vi "SV TDMS Read Function Info.vi"(8 "error in (no error)":errorcluster, 9 "channel name":string, 10 "group name":string, 11 "tdms file in":refnum<k34>) -> (0 "error out":errorcluster, 1 "channel name out":string, 2 "group name out":string, 3 "tdms file out":refnum<k34>, 4 "function info":T2 {"function type" items=["Signal"=0, "Speed"=3, "Ratio"=6, "Count"=7, "-"=9, "Level"=10, "-"=19, "Octave Spectrum"=20, "-"=29, "FFT Auto Spectrum"=30, "FFT Cross Spectrum"=40, "Frequency Response"=50, "-"=59, "Event"=90, "None"=98]; "function subtype" items=["Unscaled binary"=0, "Scaled voltage"=1, "Scaled engineering units"=2, "-"=10, "Value"=19, "DC"=11, "AC"=12, "RMS^2"=13, "RMS"=14, "Peak"=15, "Peak to peak"=16, "-"=20, "1/1 octave"=21, "1/3 octave"=22, "1/6 octave"=23, "1/12 octave"=24, "1/24 octave"=25, "-"=30, "Density"=31, "Magnitude"=32, "Phase"=33, "Real"=34, "Imaginary"=35, "Complex"=345, "Coherence"=36, "-"=90, "None"=98, "Unknown"=99]; "X-dimension" items=["Time (s)"=0, "Frequency-CB (Hz)"=1, "Frequency-CPB (Hz)"=1248, "Frequency-Arbitrary (Hz)"=2357, "Quefrency (s)"=2, "Revolutions (rev)"=3, "Order"=4, "Speed (RPM)"=11, "Speed (rad/s)"=21, "Critical Band"=31, "Critical Band Rate (Bark)"=32, "None"=98, "Index"=65535]}, 6 "LabVIEW datatype":T1 items=["String: abc"=7, "Boolean: True or False"=8, "Scalar: y"=0, "Array: Y"=1, "Waveform: t0, dt, Y, variant"=2, "Cluster: x0, dx, Y"=3, "Cluster: X, Y"=4, "Waterfall"=5, "Colormap"=6])   [LabVIEW 2017]
uses:
  <vilib>/addons/_NISVFA/_Shared subVIs/Controls/NI Function Info.ctl
  <vilib>/addons/_NISVFA/_Shared subVIs/Controls/NI Function Type.ctl
  <vilib>/addons/_NISVFA/_Shared subVIs/Controls/NI Function SubType.ctl
  <vilib>/addons/_NISVFA/_Shared subVIs/Controls/svc_X-Axis Units.ctl
  <vilib>/addons/_NISVFA/_Shared subVIs/Controls/LV Datatypes.ctl
  <vilib>/addons/_NISVFA/_Shared subVIs/Controls/NI Channel Properties.ctl
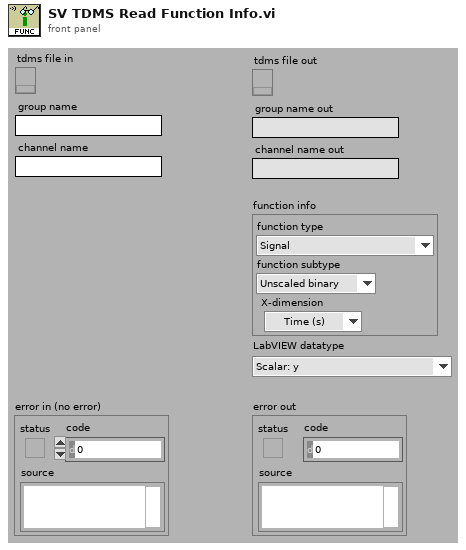
[diagram p1: front panel]
types:
  T1 = typedef "LV Datatypes.ctl" = i32
  T2 = typedef "NI Function Info.ctl" = cluster{"function type":T3, "function subtype":T4, "X-dimension":T5}
  T3 = typedef "NI Function Type.ctl" = u16
  T4 = typedef "NI Function SubType.ctl" = u16
  T5 = typedef "svc_X-Axis Units.ctl" = u16
  T6 = typedef "NI Channel Properties.ctl" = u16
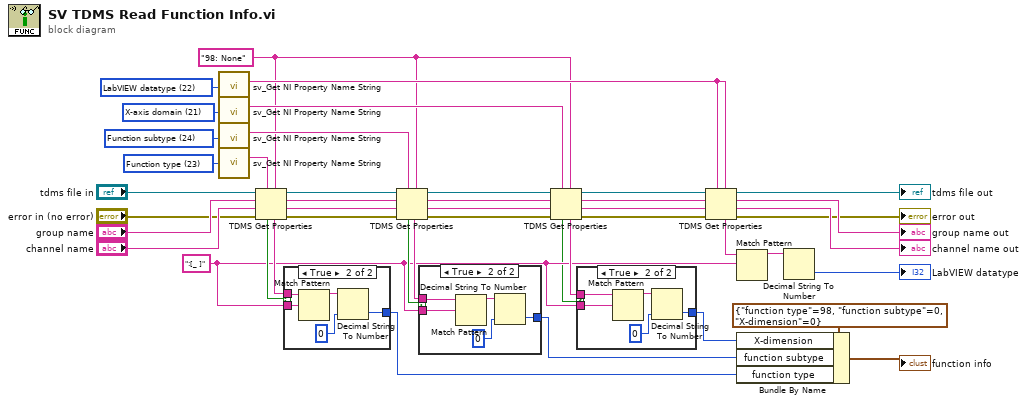
[diagram p0: block diagram]
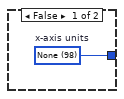
[diagram p2: hidden frame]
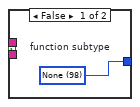
[diagram p3: hidden frame]
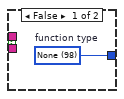
[diagram p4: hidden frame]
diagram:
  w1 = "98: None" ("data type")
  w4 = ":[_ ]" ("regular expression")
  w29 = T6 22 items=["Channel name", "Channel description", "Y-axis label", "Y-axis unit string", "X-axis label", "X-axis unit string", "x0", "dx", "Number of samples", "X channel", "Filter settled", "dB reference", "Window", "Window parameter", "Window size", "FFT size", "Peak units", "Spectrum type", "Magnitude scale", "Spectral density", "Sensor sensitivity (mV/EU)", "X-axis domain", "LabVIEW datatype"] ("property")
  w31 = T6 24 items=["Channel name", "Channel description", "Y-axis label", "Y-axis unit string", "X-axis label", "X-axis unit string", "x0", "dx", "Number of samples", "X channel", "Filter settled", "dB reference", "Window", "Window parameter", "Window size", "FFT size", "Peak units", "Spectrum type", "Magnitude scale", "Spectral density", "Sensor sensitivity (mV/EU)", "X-axis dimension", "LabVIEW datatype", "Function type", "Function subtype"] ("property")
  w32 = T6 21 items=["Channel name", "Channel description", "Y-axis label", "Y-axis unit string", "X-axis label", "X-axis unit string", "x0", "dx", "Number of samples", "X channel", "Filter settled", "dB reference", "Window", "Window parameter", "Window size", "FFT size", "Peak units", "Spectrum type", "Magnitude scale", "Spectral density", "Sensor sensitivity (mV/EU)", "X-axis domain", "LabVIEW datatype", "Function type", "Component", "Level detector"] ("property")
  w30 = T6 23 items=["Channel name", "Channel description", "Y-axis label", "Y-axis unit string", "X-axis label", "X-axis unit string", "x0", "dx", "Number of samples", "X channel", "Filter settled", "dB reference", "Window", "Window parameter", "Window size", "FFT size", "Peak units", "Spectrum type", "Magnitude scale", "Spectral density", "Sensor sensitivity (mV/EU)", "X-axis domain", "LabVIEW datatype", "Function type", "Component", "Level detector"] ("property")
  n1 = call <vilib>:"sv_Get NI Property Name String.vi"("property"=w29) -> ("TDMS property name"=w17:string)  [unwired: 13 in, 1 out]
  n2 = call <vilib>:"sv_Get NI Property Name String.vi"("property"=w32) -> ("TDMS property name"=w18:string)  [unwired: 13 in, 1 out]
  n3 = call <vilib>:"sv_Get NI Property Name String.vi"("property"=w31) -> ("TDMS property name"=w19:string)  [unwired: 13 in, 1 out]
  n4 = call <vilib>:"sv_Get NI Property Name String.vi"("property"=w30) -> ("TDMS property name"=w20:string)  [unwired: 13 in, 1 out]
  n5 = TDMS Get Properties(5:w1, 7:w20, 8:"error in (no error)", 9:"channel name", 10:"group name", 11:"tdms file in") -> (0:w37:errorcluster, 1:w38:string, 2:w39:string, 3:w40:refnum<k34>, 4:w16:string, 6:w10:bool)
  n6 = case shown="True" w10 {
    tunnel: w16 -> [_ w49]
    tunnel: [w45 w48] -> w14
    tunnel: w4 -> [_ w47]
    frame False {
      w45 = T3 98 items=["Signal"=0, "Speed"=3, "Ratio"=6, "Count"=7, "-"=9, "Level"=10, "-"=19, "Octave Spectrum"=20, "-"=29, "FFT Auto Spectrum"=30, "FFT Cross Spectrum"=40, "Frequency Response"=50, "-"=59, "Event"=90, "None"=98]  # function type
    }
    frame True {
      n7 = Match Pattern(string=w49, regular expression=w47) -> (before substring=w50:string)  [unwired: 1 in, 3 out]
      n8 = Decimal String To Number(string=w50, default (0L)=u16 0 ("default (0 I32)")) -> (number=w48:u16)  [unwired: 1 in, 1 out]
    }
  }
  n9 = TDMS Get Properties(5:w1, 7:w19, 8:w37, 9:w38, 10:w39, 11:w40) -> (0:w44:errorcluster, 1:w43:string, 2:w42:string, 3:w41:refnum<k34>, 4:w7:string, 6:w8:bool)
  n10 = case shown="True" w8 {
    tunnel: w7 -> [_ w55]
    tunnel: [w51 w54] -> w6
    tunnel: w4 -> [_ w53]
    frame False {
      w51 = T4 98 items=["Unscaled binary"=0, "Scaled voltage"=1, "Scaled engineering units"=2, "-"=10, "Value"=19, "DC"=11, "AC"=12, "RMS^2"=13, "RMS"=14, "Peak"=15, "Peak to peak"=16, "-"=20, "1/1 octave"=21, "1/3 octave"=22, "1/6 octave"=23, "1/12 octave"=24, "1/24 octave"=25, "-"=30, "Density"=31, "Magnitude"=32, "Phase"=33, "Real"=34, "Imaginary"=35, "Complex"=345, "Coherence"=36, "-"=90, "None"=98, "Unknown"=99]  # function subtype
    }
    frame True {
      n11 = Match Pattern(string=w55, regular expression=w53) -> (before substring=w56:string)  [unwired: 1 in, 3 out]
      n12 = Decimal String To Number(string=w56, default (0L)=u16 0 ("default (0 I32)")) -> (number=w54:u16)  [unwired: 1 in, 1 out]
    }
  }
  n13 = TDMS Get Properties(5:w1, 7:w18, 8:w44, 9:w43, 10:w42, 11:w41) -> (0:w22:errorcluster, 1:w28:string, 2:w27:string, 3:w26:refnum<k34>, 4:w5:string, 6:w2:bool)
  n14 = case shown="True" w2 {
    tunnel: [w57 w61] -> w3
    tunnel: w5 -> [_ w59]
    tunnel: w4 -> [_ w58]
    frame False {
      w57 = T5 98 items=["Time (s)"=0, "Frequency-CB (Hz)"=1, "Frequency-CPB (Hz)"=1248, "Frequency-Arbitrary (Hz)"=2357, "Quefrency (s)"=2, "Revolutions (rev)"=3, "Order"=4, "Speed (RPM)"=11, "Speed (rad/s)"=21, "Critical Band"=31, "Critical Band Rate (Bark)"=32, "None"=98, "Index"=65535]  # x-axis units
    }
    frame True {
      n15 = Match Pattern(string=w59, regular expression=w58) -> (before substring=w62:string)  [unwired: 1 in, 3 out]
      n16 = Decimal String To Number(string=w62, default (0L)=u16 0 ("default (0 I32)")) -> (number=w61:u16)  [unwired: 1 in, 1 out]
    }
  }
  n17 = TDMS Get Properties(5:w17, 7:w17, 8:w22, 9:w28, 10:w27, 11:w26) -> (0:→"error out":errorcluster, 1:→"channel name out":string, 2:→"group name out":string, 3:→"tdms file out":refnum<k34>, 4:w12:string)  [unwired: 1 out]
  n18 = Match Pattern(string=w12, regular expression=w4) -> (before substring=w13:string)  [unwired: 1 in, 3 out]
  n19 = Bundle By Name(cluster=T2 {"function type"=98, "function subtype"=0, "X-dimension"=0}, "X-dimension"=w3, "function subtype"=w6, "function type"=w14) -> (→"function info":T2)
  n20 = Decimal String To Number(string=w13) -> (number=→"LabVIEW datatype":i32)  [unwired: 2 in, 1 out]
